vi "Calibration_Hall_full.vi"(9 "Reset Field":dbl, 10 "Min Field":dbl=0.5 format="%#_13g", 11 "Max Field":dbl=0.5 format="%#_13g") -> (2 "Calibration Curve":cluster{dbl[], "Best Linear Fit":dbl[]}[](graph)=[{[0.0, 0.005, 0.01, 0.015, 0.02, 0.025, 0.03, 0.035, 0.04, 0.045, 0.05, 0.055, 0.06, 0.065, 0.07, 0.075, 0.08, 0.085, 0.09, 0.095, 0.1, 0.105, 0.11, 0.115, 0.12, 0.125, 0.13, 0.135, 0.14, 0.145, 0.15, 0.155, 0.16, 0.165, 0.17, 0.175, 0.18, 0.185, 0.19, 0.195, 0.2, 0.205, 0.21, 0.215, 0.22, 0.225, 0.23, 0.235, 0.24, 0.245, 0.25, 0.255, 0.26, 0.265, 0.27, 0.275, 0.28, 0.285, 0.29, 0.295, 0.3, 0.305, 0.31, 0.315, 0.32, 0.325, 0.33, 0.335, 0.34, 0.345, 0.35, 0.355, 0.36, 0.365, 0.37, 0.375, 0.38, 0.385, 0.39, 0.395, 0.4, 0.405, 0.41, 0.415, 0.42, 0.425, 0.43, 0.435, 0.44, 0.445, 0.45, 0.455, 0.46, 0.465, 0.47, 0.475, 0.48, 0.485, 0.49, 0.495, 0.5], "Best Linear Fit"=[-1.7e-06, 1.18e-05, 3.66e-05, 6.17e-05, 9.39e-05, 0.000122, 0.0001511, 0.0001781, 0.0002061, 0.0002355, 0.0002616, 0.0002895, 0.0003184, 0.0003446, 0.0003689, 0.0003958, 0.0004207, 0.0004464, 0.0004684, 0.0004953, 0.0005218, 0.0005459, 0.0005692, 0.0005897, 0.0006131, 0.0006347, 0.0006589, 0.0006834, 0.0007035, 0.0007249, 0.0007465, 0.000765, 0.0007858, 0.0008103, 0.0008302, 0.0008467, 0.000868, 0.0008855, 0.0009079, 0.0009248, 0.0009452, 0.0009633, 0.0009828, 0.0009992, 0.0010189, 0.0010338, 0.001054, 0.0010692, 0.0010858, 0.0011036, 0.0011162, 0.0011356, 0.0011502, 0.0011643, 0.0011834, 0.0011985, 0.0012131, 0.0012277, 0.0012423, 0.0012571, 0.0012691, 0.0012827, 0.0012976, 0.001313, 0.0013264, 0.0013388, 0.0013518, 0.0013638, 0.0013782, 0.0013909, 0.0014035, 0.0014175, 0.0014295, 0.0014407, 0.0014538, 0.0014641, 0.0014752, 0.0014861, 0.0014978, 0.0015081, 0.0015203, 0.001532, 0.0015422, 0.0015526, 0.001563, 0.0015754, 0.0015844, 0.0015955, 0.0016056, 0.001614, 0.0016239, 0.0016342, 0.0016457, 0.0016542, 0.0016635, 0.001674, 0.001681, 0.0016886, 0.0016986, 0.0017063, 0.0017155]}, {[0.0, 0.005, 0.01, 0.015, 0.02, 0.025, 0.03, 0.035, 0.04, 0.045, 0.05, 0.055, 0.06, 0.065, 0.07, 0.075, 0.08, 0.085, 0.09, 0.095, 0.1, 0.105, 0.11, 0.115, 0.12, 0.125, 0.13, 0.135, 0.14, 0.145, 0.15, 0.155, 0.16, 0.165, 0.17, 0.175, 0.18, 0.185, 0.19, 0.195, 0.2, 0.205, 0.21, 0.215, 0.22, 0.225, 0.23, 0.235, 0.24, 0.245, 0.25, 0.255, 0.26, 0.265, 0.27, 0.275, 0.28, 0.285, 0.29, 0.295, 0.3, 0.305, 0.31, 0.315, 0.32, 0.325, 0.33, 0.335, 0.34, 0.345, 0.35, 0.355, 0.36, 0.365, 0.37, 0.375, 0.38, 0.385, 0.39, 0.395, 0.4, 0.405, 0.41, 0.415, 0.42, 0.425, 0.43, 0.435, 0.44, 0.445, 0.45, 0.455, 0.46, 0.465, 0.47, 0.475, 0.48, 0.485, 0.49, 0.495, 0.5], "Best Linear Fit"=[-1.7e-06, 1.18e-05, 3.66e-05, 6.17e-05, 9.39e-05, 0.000122, 0.0001511, 0.0001781, 0.0002061, 0.0002355, 0.0002616, 0.0002895, 0.0003184, 0.0003446, 0.0003689, 0.0003958, 0.0004207, 0.0004464, 0.0004684, 0.0004953, 0.0005218, 0.0005459, 0.0005692, 0.0005897, 0.0006131, 0.0006347, 0.0006589, 0.0006834, 0.0007035, 0.0007249, 0.0007465, 0.000765, 0.0007858, 0.0008103, 0.0008302, 0.0008467, 0.000868, 0.0008855, 0.0009079, 0.0009248, 0.0009452, 0.0009633, 0.0009828, 0.0009992, 0.0010189, 0.0010338, 0.001054, 0.0010692, 0.0010858, 0.0011036, 0.0011162, 0.0011356, 0.0011502, 0.0011643, 0.0011834, 0.0011985, 0.0012131, 0.0012277, 0.0012423, 0.0012571, 0.0012691, 0.0012827, 0.0012976, 0.001313, 0.0013264, 0.0013388, 0.0013518, 0.0013638, 0.0013782, 0.0013909, 0.0014035, 0.0014175, 0.0014295, 0.0014407, 0.0014538, 0.0014641, 0.0014752, 0.0014861, 0.0014978, 0.0015081, 0.0015203, 0.001532, 0.0015422, 0.0015526, 0.001563, 0.0015754, 0.0015844, 0.0015955, 0.0016056, 0.001614, 0.0016239, 0.0016342, 0.0016457, 0.0016542, 0.0016635, 0.001674, 0.001681, 0.0016886, 0.0016986, 0.0017063, 0.0017155]}], 3 "Calibration Curve Data":dbl[][](array[numeric])=[[0.0, 0.005, 0.01, 0.015, 0.02, 0.025, 0.03, 0.035, 0.04, 0.045, 0.05, 0.055, 0.06, 0.065, 0.07, 0.075, 0.08, 0.085, 0.09, 0.095, 0.1, 0.105, 0.11, 0.115, 0.12, 0.125, 0.13, 0.135, 0.14, 0.145, 0.15, 0.155, 0.16, 0.165, 0.17, 0.175, 0.18, 0.185, 0.19, 0.195, 0.2, 0.205, 0.21, 0.215, 0.22, 0.225, 0.23, 0.235, 0.24, 0.245, 0.25, 0.255, 0.26, 0.265, 0.27, 0.275, 0.28, 0.285, 0.29, 0.295, 0.3, 0.305, 0.31, 0.315, 0.32, 0.325, 0.33, 0.335, 0.34, 0.345, 0.35, 0.355, 0.36, 0.365, 0.37, 0.375, 0.38, 0.385, 0.39, 0.395, 0.4, 0.405, 0.41, 0.415, 0.42, 0.425, 0.43, 0.435, 0.44, 0.445, 0.45, 0.455, 0.46, 0.465, 0.47, 0.475, 0.48, 0.485, 0.49, 0.495, 0.5], [-1.7e-06, 1.18e-05, 3.66e-05, 6.17e-05, 9.39e-05, 0.000122, 0.0001511, 0.0001781, 0.0002061, 0.0002355, 0.0002616, 0.0002895, 0.0003184, 0.0003446, 0.0003689, 0.0003958, 0.0004207, 0.0004464, 0.0004684, 0.0004953, 0.0005218, 0.0005459, 0.0005692, 0.0005897, 0.0006131, 0.0006347, 0.0006589, 0.0006834, 0.0007035, 0.0007249, 0.0007465, 0.000765, 0.0007858, 0.0008103, 0.0008302, 0.0008467, 0.000868, 0.0008855, 0.0009079, 0.0009248, 0.0009452, 0.0009633, 0.0009828, 0.0009992, 0.0010189, 0.0010338, 0.001054, 0.0010692, 0.0010858, 0.0011036, 0.0011162, 0.0011356, 0.0011502, 0.0011643, 0.0011834, 0.0011985, 0.0012131, 0.0012277, 0.0012423, 0.0012571, 0.0012691, 0.0012827, 0.0012976, 0.001313, 0.0013264, 0.0013388, 0.0013518, 0.0013638, 0.0013782, 0.0013909, 0.0014035, 0.0014175, 0.0014295, 0.0014407, 0.0014538, 0.0014641, 0.0014752, 0.0014861, 0.0014978, 0.0015081, 0.0015203, 0.001532, 0.0015422, 0.0015526, 0.001563, 0.0015754, 0.0015844, 0.0015955, 0.0016056, 0.001614, 0.0016239, 0.0016342, 0.0016457, 0.0016542, 0.0016635, 0.001674, 0.001681, 0.0016886, 0.0016986, 0.0017063, 0.0017155]])   [LabVIEW 2015]
panel:
  in  "stop 2":bool
  in  "dB":dbl=0.005
  in  "Dwell Time (ms)":u32=1000
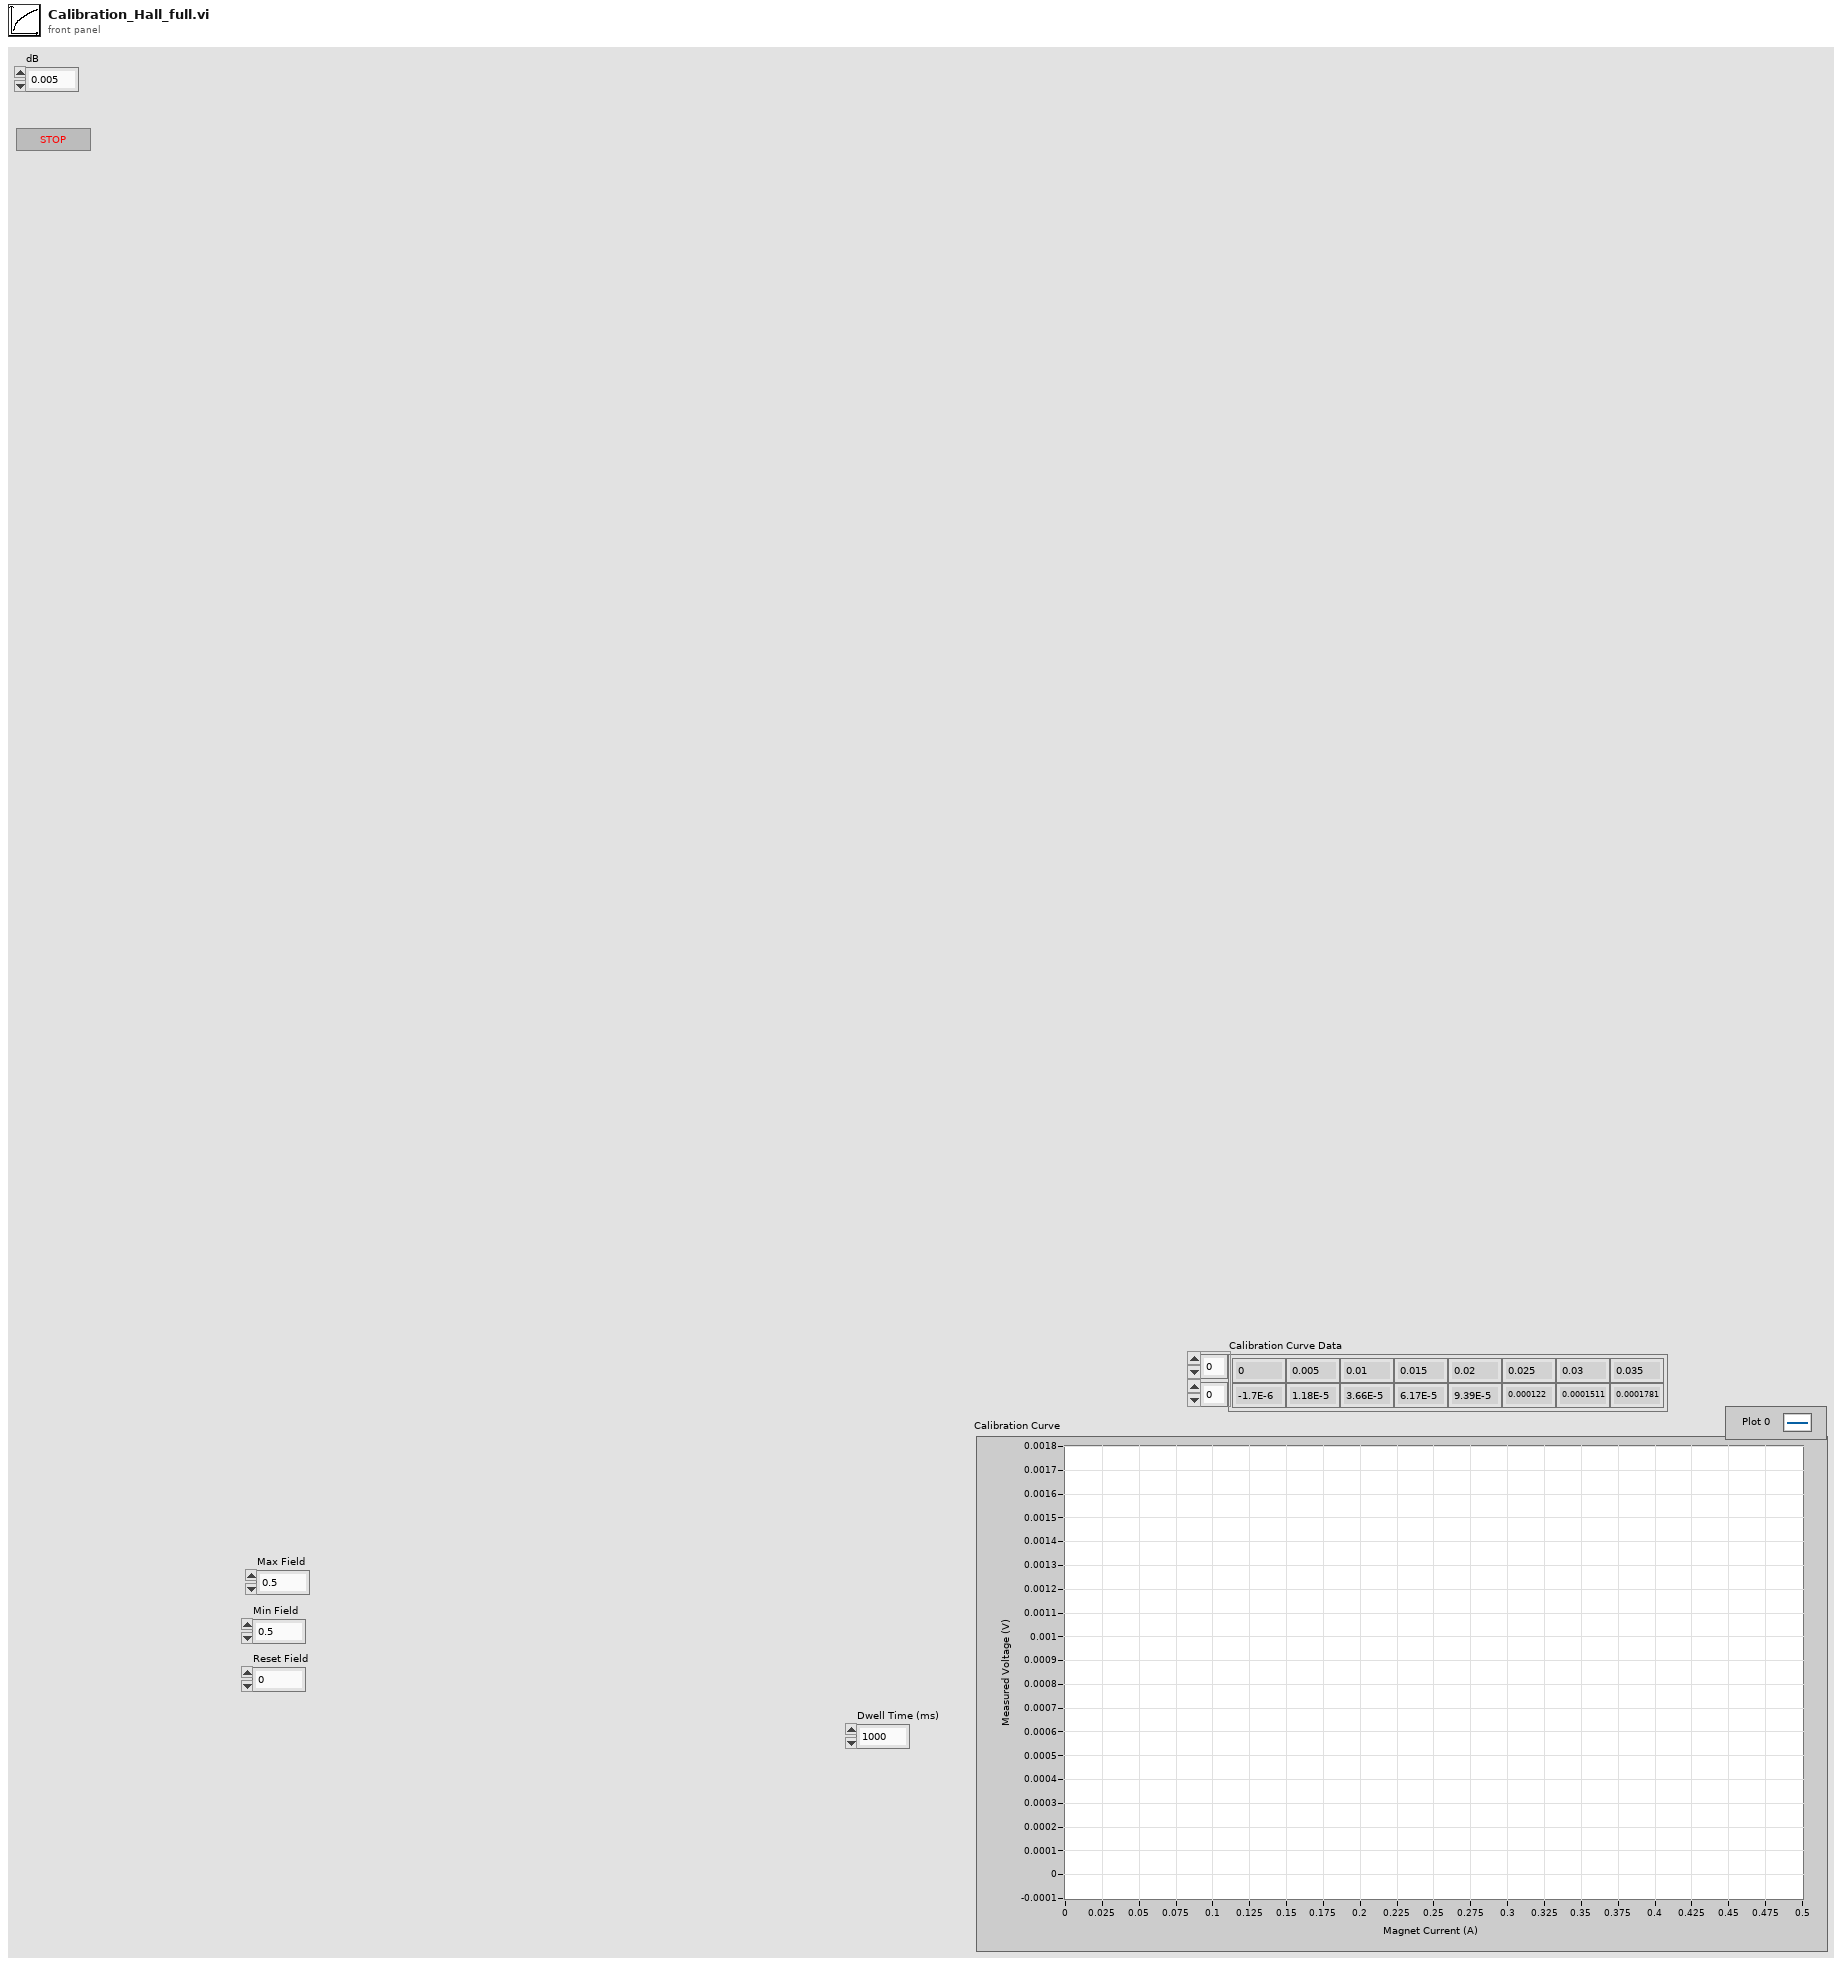
[diagram p1: front panel]
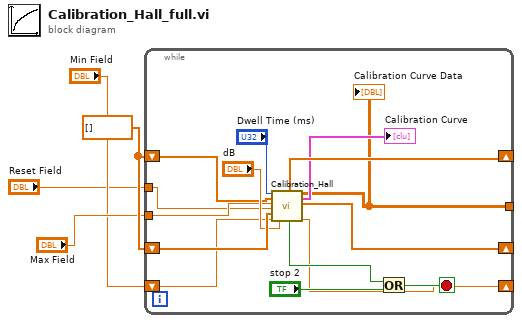
[diagram p0: block diagram]
diagram:
  w4 = dbl[] []
  n1 = while {
    shift-right: [w15] -> _
    shift-left: w4 -> [w16]
    shift-right: [w9] -> _
    shift-left: w4 -> [w10]
    shift-right: [w12] -> _
    shift-left: "Min Field" -> [w11]
    tunnel: [w7] -> _
    tunnel: "Max Field" -> [w6]
    tunnel: "Reset Field" -> [w5]
    stop <- w17 stop-if-true
    n2 = call "Calibration_Hall.vi"("Dwell Time (ms)"="Dwell Time (ms)", "R array in (V)"=w10, "Max Field"=w6, "Reset Field"=w5, "B array in (T)"=w16, "Set Field (T)"=w11, "dB"="dB") -> ("R array out (V)"=w9:dbl[], "Ready?"=w19:bool, 14:"Calibration Curve"=w7:dbl[][], 15:"Calibration Curve"=→"Calibration Curve":cluster{dbl[], dbl[]}[], "B array Out"=w15:dbl[], "Set Field out"=w12:dbl)  [unwired: 7 in]
    "Calibration Curve Data" <- w7
    n3 = Or(x=w19, y="stop 2") -> (x .or. y?=w17:bool)
  }
